vi "login.vi"() -> (2 "correct":bool)   [LabVIEW 2014]
panel:
  in  "?":bool
  in  "password":string
  in  "username":string
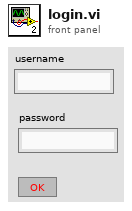
[diagram p1: front panel]
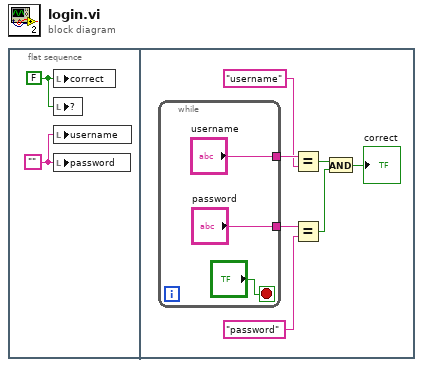
[diagram p0: block diagram]
diagram:
  n1 = flat-sequence {
    frame #0 {
      w1 = FALSE
      w2 = ""
      n2 = local write "correct"(w1) -> ()
      n3 = local write item#3(w1) -> ()
      n4 = local write "username"(w2) -> ()
      n5 = local write "password"(w2) -> ()
    }
    frame #1 {
      n6 = while {
        tunnel: ["username"] -> w7
        tunnel: ["password"] -> w5
        stop <- "?" stop-if-true
      }
      n7 = Equal?(x=w7, y="username") -> (x = y?=w8:bool)
      n8 = Equal?(x=w5, y="password") -> (x = y?=w9:bool)
      n9 = And(x=w8, y=w9) -> (x .and. y?=→"correct":bool)
    }
  }
